vi "Set Report Header Text.vi"(4 "header placement":enum16{"Top of Document", "Append to Body"}(ring), 6 "HTML header size":enum16{"H1", "H2", "H3", "H4", "H5", "H6", "H7"}(ring)=enum."H3", 7 "left header text":string, 8 "error in (no error)":errorcluster, 9 "right header text":string, 10 "center header text":string, 11 "report in":T1) -> (0 "error out":errorcluster, 3 "report out":T1)   [LabVIEW 2020]
doc: "Sets the text of the report header."
uses:
  <vilib>/Utility/NIReport.llb/Generate Report Object Reference.ctl
  <vilib>/Utility/NIReport.llb/NI_report.lvclass
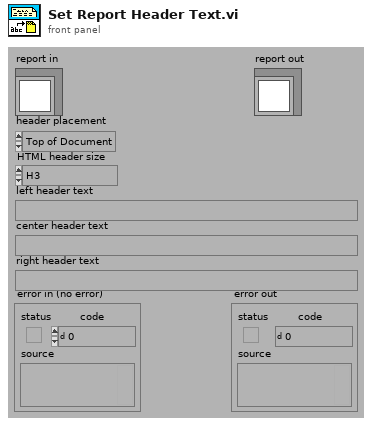
[diagram p1: front panel]
types:
  T1 = typedef "Generate Report Object Reference.ctl" = refnum<class "NI_report.lvclass">
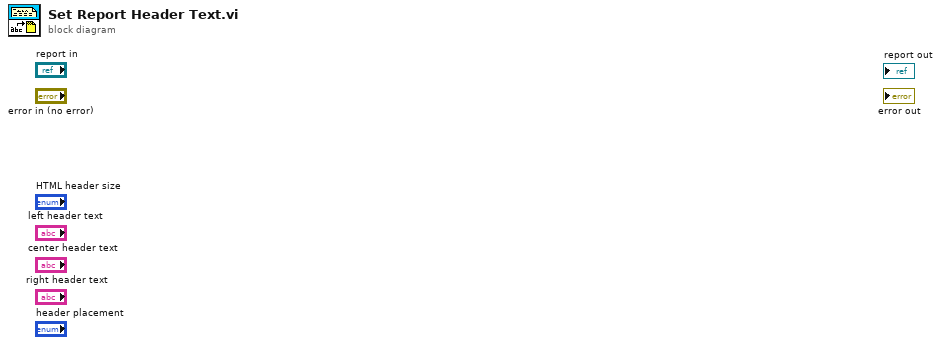
[diagram p0: block diagram]
diagram:
